vi "JKISM+ Worker Module.vi"(7 "Name":string="A") -> ()   [LabVIEW 2014]
uses:
  user.lib/_NEVSTOP/JKI State Machine ++/JKI-State-Machine-Plus.lvlib
panel:
  out "From Who":string
  out "Argument - State":string
  out "Arguments":string
  out "Current State":string
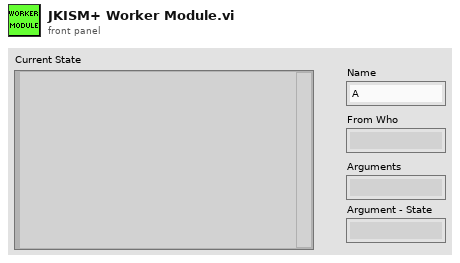
[diagram p1: front panel]
types:
  T1 = enum32{"Invalid", "Standard", "Closed", "Hidden", "Minimized", "Maximized"}
  T2 = enum32{"invalid app kind", "Development System", "Run Time System", "Student Edition", "Embedded LabVIEW", "Evaluation", "Custom"}
  T3 = cluster{"Core":cluster{"Current VI Reference":refnum<vi>, "Close Panel on Exit?":bool}, "Your Boolean data":bool, "Your string data":string}
  T4 = cluster{"Current VI Reference":refnum<vi>, "Close Panel on Exit?":bool}
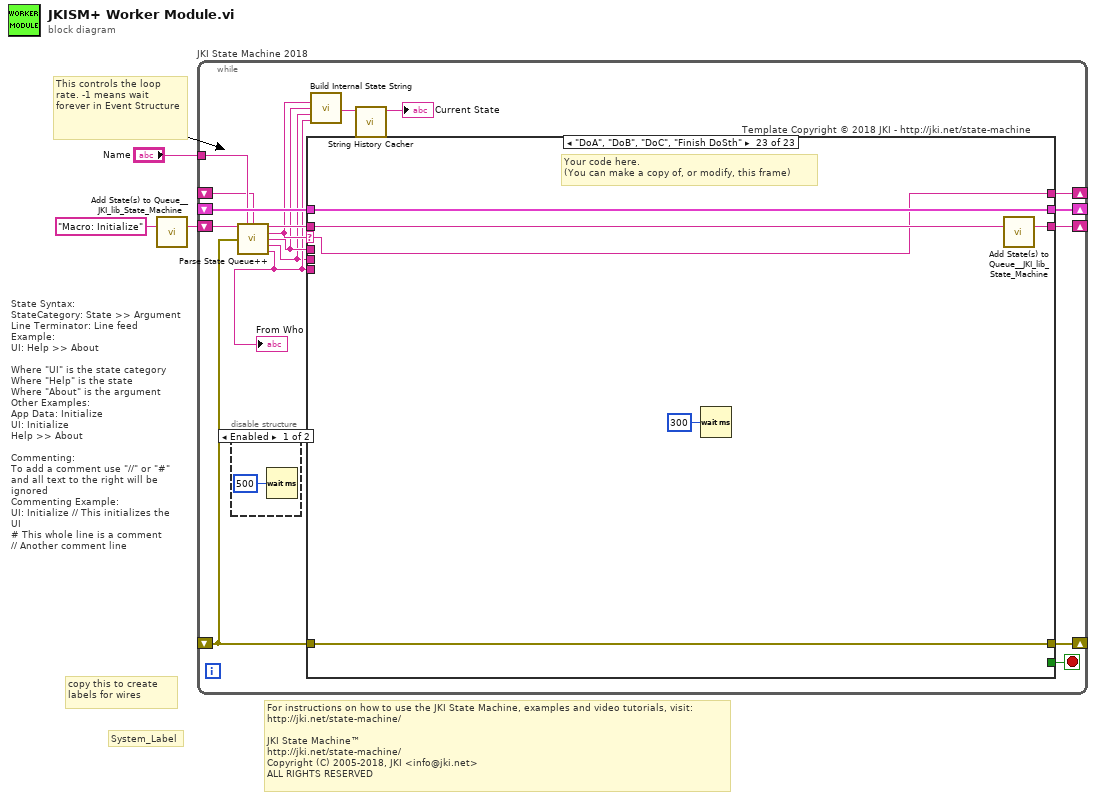
[diagram p0: block diagram]
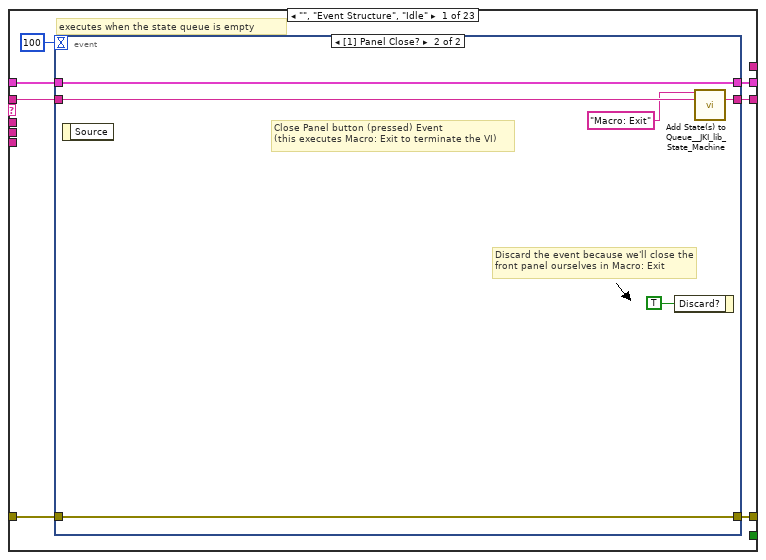
[diagram p3: hidden frame]
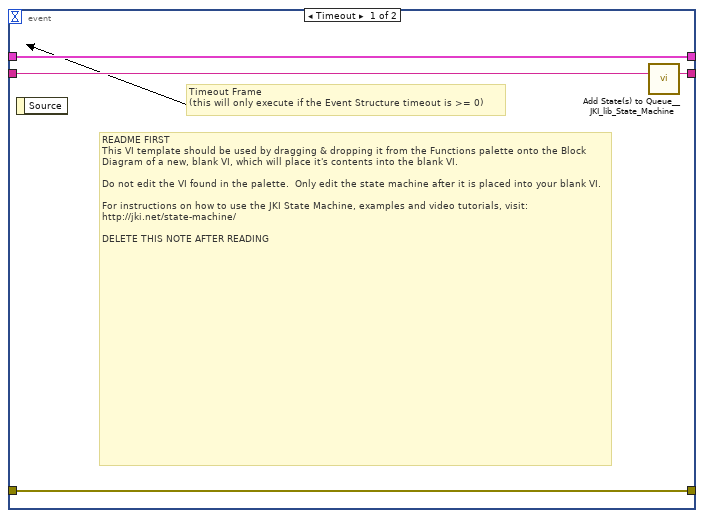
[diagram p4: hidden frame]
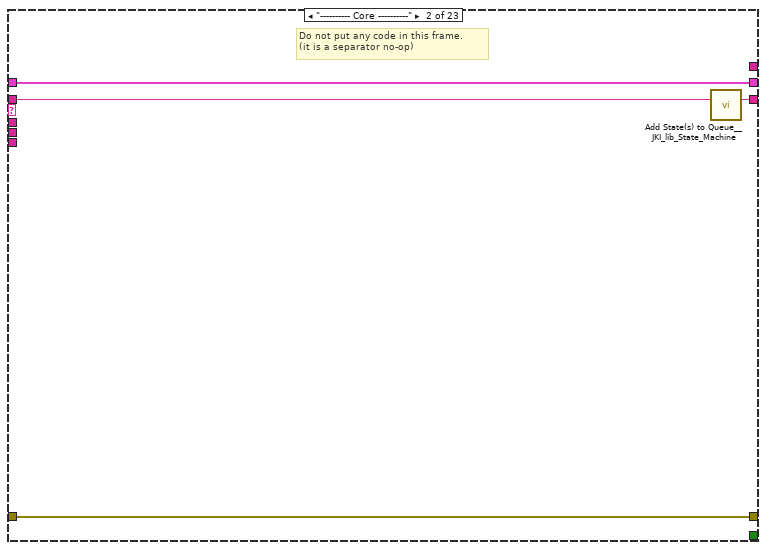
[diagram p5: hidden frame]
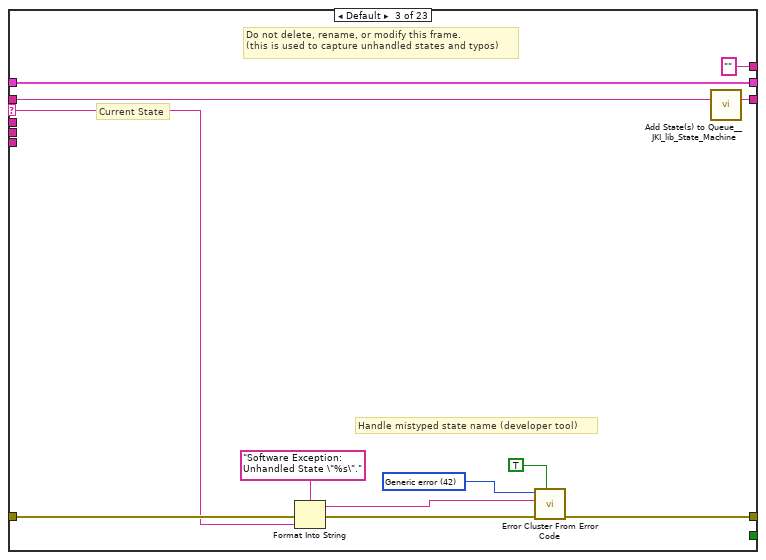
[diagram p6: hidden frame]
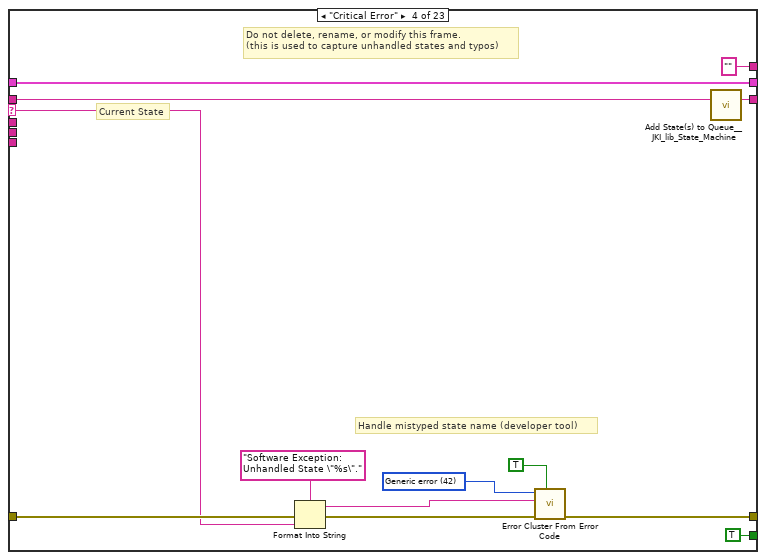
[diagram p7: hidden frame]
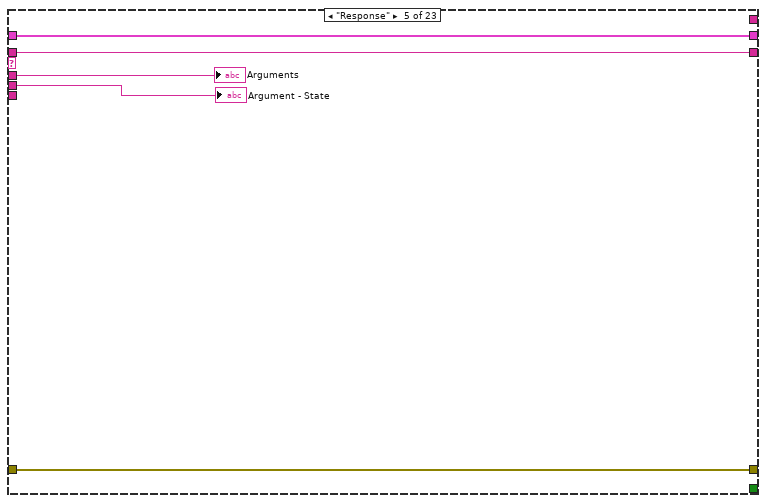
[diagram p8: hidden frame]
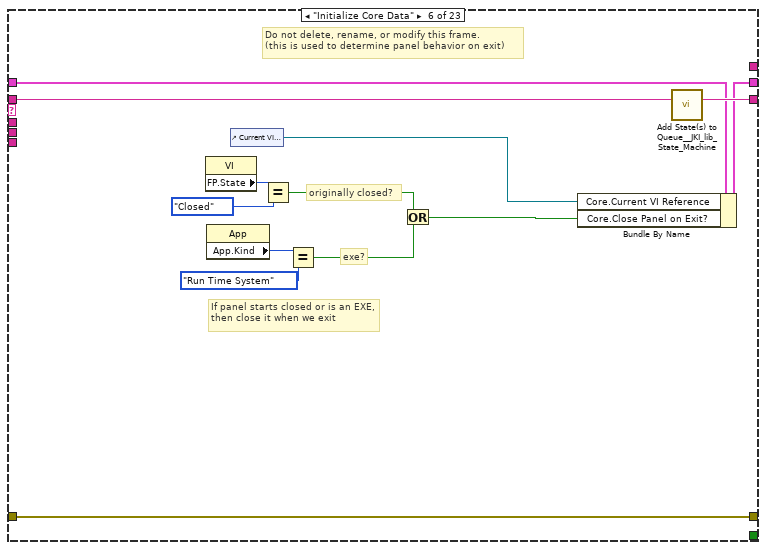
[diagram p9: hidden frame]
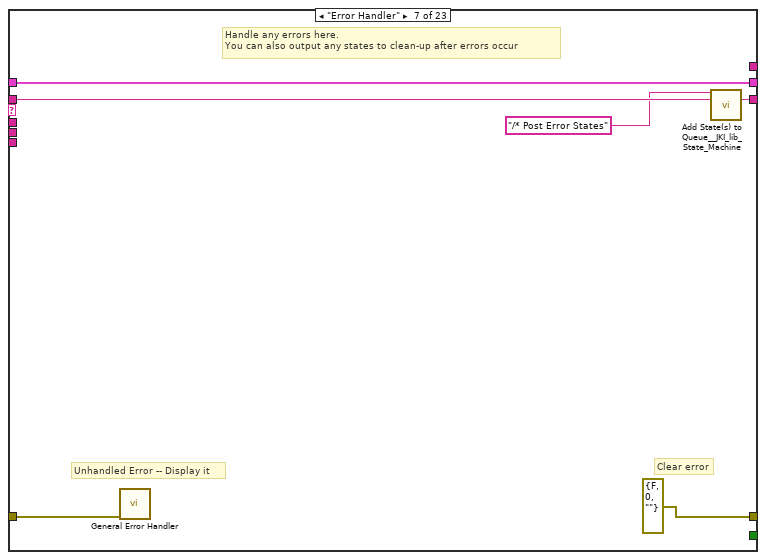
[diagram p10: hidden frame]
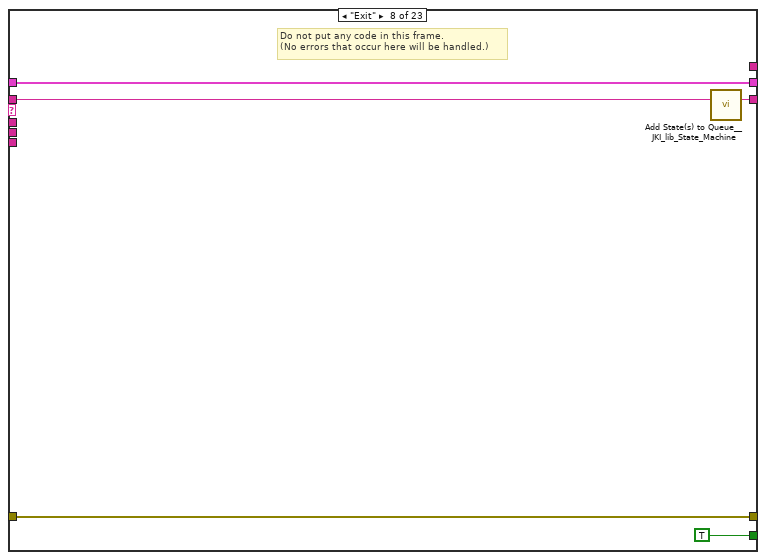
[diagram p11: hidden frame]
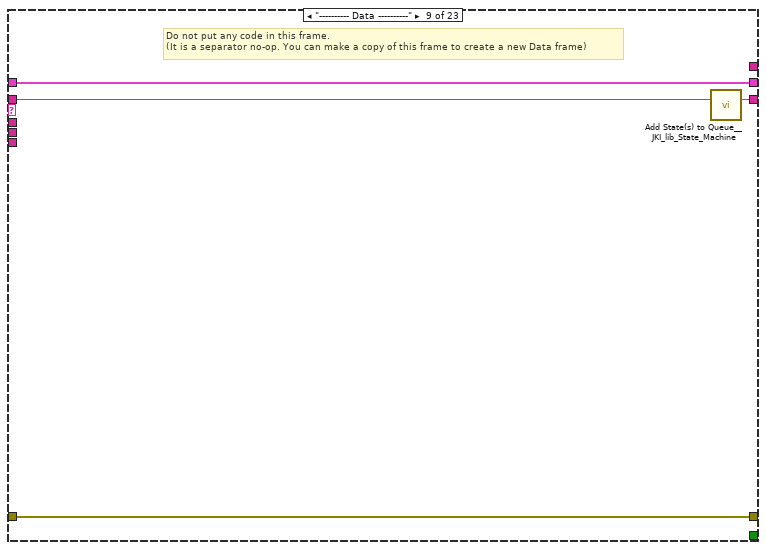
[diagram p12: hidden frame]
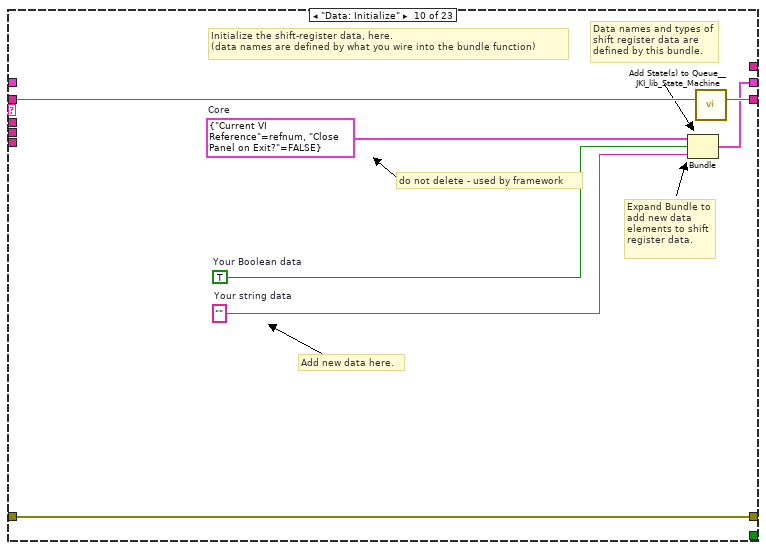
[diagram p13: hidden frame]
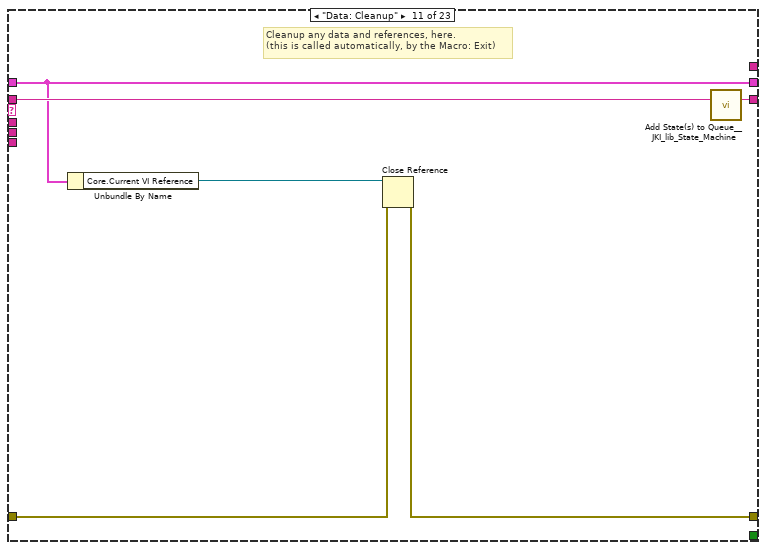
[diagram p14: hidden frame]
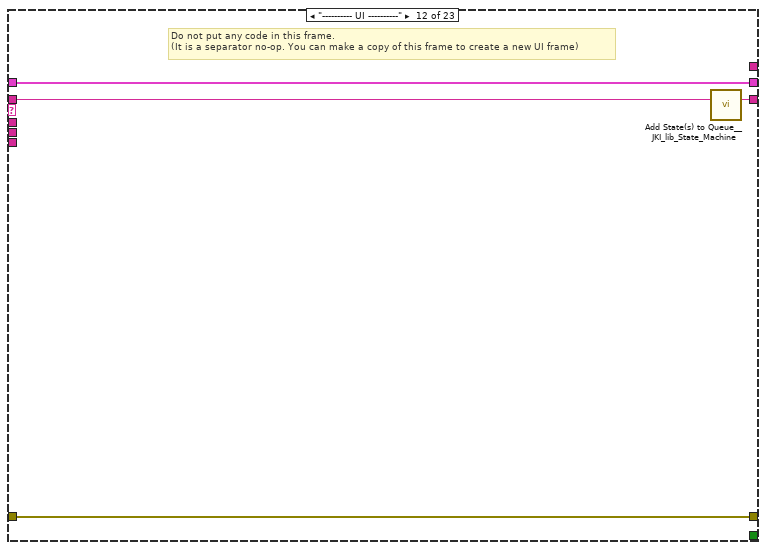
[diagram p15: hidden frame]
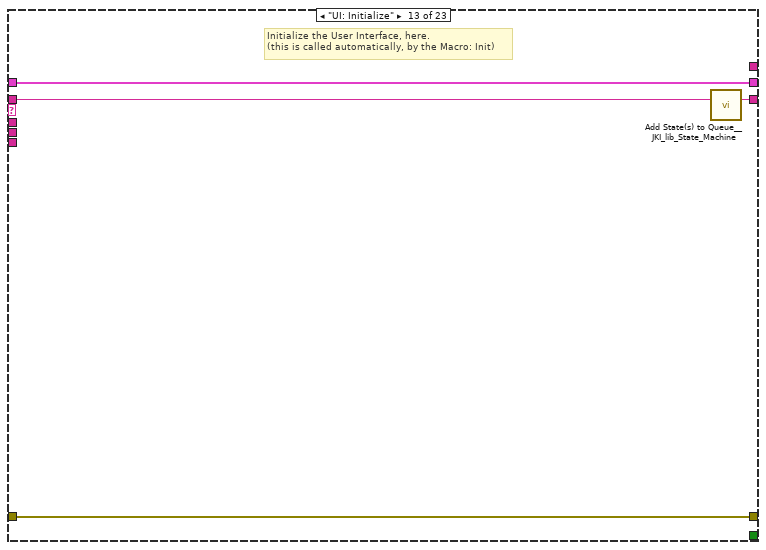
[diagram p16: hidden frame]
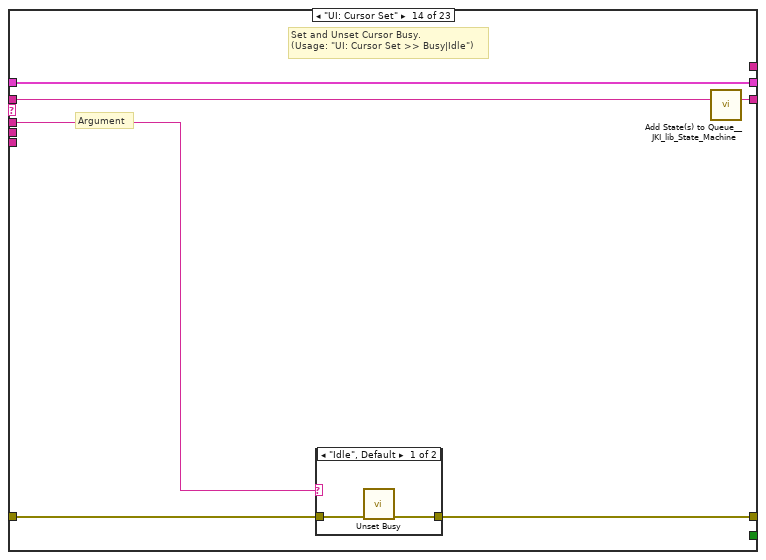
[diagram p17: hidden frame]
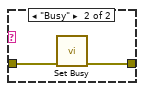
[diagram p18: hidden frame]
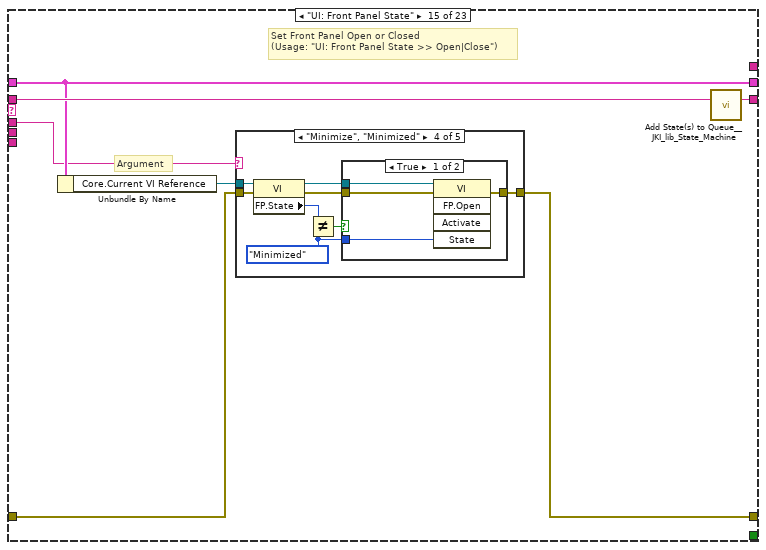
[diagram p19: hidden frame]
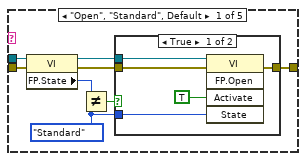
[diagram p20: hidden frame]
diagram:
  # "For instructions on how to use the JKI State Machine, examples and video tutorials, visit:\nhttp://jki.net/state-machine/\n\nJKI State Machine™\nhttp://jki.net/state-machine/\nCopyright (C) 2005-2018, JKI <info@jki.net>\nALL RIGHTS RESERVED"
  # "State Syntax:\nStateCategory: State >> Argument\nLine Terminator: Line feed\nExample:\nUI: Help >> About\n\nWhere \"UI\" is the state category\nWhere \"Help\" is the state\nWhere \"About\" is the argument\nOther Examples:\nApp Data: Initialize\nUI: Initialize\nHelp >> About\n\nCommenting:\nTo add a comment use \"//\" or \"#\" and all text to the right will be ignored\nCommenting Example:\nUI: Initialize // This initializes the UI\n# This whole line is a comment\n// Another comment line"
  # "copy this to create labels for wires"
  # "This controls the loop rate. -1 means wait forever in Event Structure"
  # "System_Label"
  n1 = call <vilib>:"Add State(s) to Queue__JKI_lib_State_Machine.vi"("State(s) in (\"\")"="Macro: Initialize") -> ("States Out"=w3:string)  [unwired: 14 in]
  n2 = while "JKI State Machine 2018" {
    shift-right: [w15] -> _
    shift-left: _ -> [w14]
    shift-right: [w18] -> _
    shift-left: _ -> [w13]
    shift-right: [w17] -> _
    shift-left: w3 -> [w19]
    tunnel: "Name" -> [w12]
    shift-right: [w5] -> _
    shift-left: _ -> [w4]
    stop <- w16 stop-if-true
    # "Template Copyright © 2018 JKI - http://jki.net/state-machine"
    n3 = disable-structure shown="Enabled" {
      frame Enabled {
        n4 = Wait (ms)(milliseconds to wait=u32 500) -> ()  [unwired: 1 out]
      }
      frame Disabled {
      }
    }
    n5 = call "Parse State Queue++.vi"("State Queue"=w19, "Name(\"\" to use uuid)"=w12, "Response Arguments"=w4, "Error In (no error)"=w13) -> ("Remaining States"=w20:string, "Current State"=w9:string, "Arguments"=w8:string, "Argument - State"=w6:string, "From Who"=w7:string)  [unwired: 7 in]
    "From Who" <- w7
    n6 = case shown="\"DoA\", \"DoB\", \"DoC\", \"Finish DoSth\"" w9 {
      selector: w9 -> [_ _ w44 w57 _ _ _ _ _ _ _ _ _ _ _ _ _ _ _ _ _ _ w240]
      tunnel: w20 -> [w28 w42 w48 w61 w72 w85 w91 w96 w100 w107 w113 w117 w121 w127 w138 w207 w212 w215 w227 w231 w235 w239 w245]
      tunnel: w8 -> [_ _ _ _ w69 _ _ _ _ _ _ _ _ w122 w132 _ _ _ _ _ _ _ _]
      tunnel: w14 -> [w26 w39 w46 w59 w71 w78 w88 w94 w97 _ w108 w114 w119 w125 w134 w204 w209 w217 w224 w228 w232 w236 w242]
      tunnel: [w25 w40 w50 w63 w70 w82 errorcluster {"status"=FALSE, "code"=0, "source"=""} ("error out") w93 w98 w104 w109 w115 w118 w123 w135 w205 w210 w213 w225 w229 w233 w237 w243] -> w18
      tunnel: w13 -> [w24 w40 w49 w62 w70 w82 w87 w93 w98 w104 w110 w115 w118 w124 w136 w205 w210 w213 w225 w229 w233 w237 w243]
      tunnel: [w27 w41 w47 w60 w72 w84 w90 w95 w99 w106 w112 w116 w120 w126 w137 w206 w211 w216 w226 w230 w234 w238 w244] -> w17
      tunnel: [_ _ _ TRUE _ _ _ TRUE _ _ _ _ _ _ _ _ _ _ _ _ _ _ _] -> w16
      tunnel: [w23 w39 w46 w59 w71 w83 w88 w94 w97 w105 w108 w114 w119 w125 w134 w204 w209 w217 w224 w228 w232 w236 w242] -> w15
      tunnel: w7 -> [_ _ _ _ _ _ _ _ _ _ _ _ _ _ _ _ _ _ _ _ _ _ _]
      tunnel: w6 -> [_ _ _ _ w68 _ _ _ _ _ _ _ _ _ _ _ _ _ _ _ _ _ _]
      tunnel: [_ _ "" ("Name") "" ("Name") _ _ _ _ _ _ _ _ _ _ _ _ _ _ _ _ _ _ w240] -> w5
      frame "", "Event Structure", "Idle" {
        # "executes when the state queue is empty"
        n7 = event shown="[1] Panel Close?" {
          selector: _ -> [_ _]
          dyn-events: _ -> [_ _]
          timeout: 100 ("Timeout") -> [_ _]
          tunnel: w28 -> [w32 w38]
          tunnel: [w31 w37] -> w27
          tunnel: w26 -> [w29 w35]
          tunnel: [w30 w36] -> w25
          tunnel: w24 -> [w30 w36]
          tunnel: [w29 w35] -> w23
          event Timeout {
            # "README FIRST\nThis VI template should be used by dragging & dropping it from the Functions palette onto the Block Diagram of a new, blank VI, which will place it's contents into the blank VI.\n\nDo not edit the VI found in the palette.  Only edit the state machine after it is placed into your blank VI.\n\nFor instructions on how to use the JKI State Machine, examples and video tutorials, visit:\nhttp://jki.net/state-machine/\n\nDELETE THIS NOTE AFTER READING"
            # "Timeout Frame\n(this will only execute if the Event Structure timeout is >= 0)"
            n8 = event-data() -> ()  [unwired: 1 in, 1 out]
            n9 = call <vilib>:"Add State(s) to Queue__JKI_lib_State_Machine.vi"("State(s) in (\"\")"=w32) -> ("States Out"=w31:string)  [unwired: 14 in]
          }
          event Panel Close? {
            # "Discard the event because we'll close the front panel ourselves in Macro: Exit"
            # "Close Panel button (pressed) Event\n(this executes Macro: Exit to terminate the VI)"
            n10 = event-data() -> ()  [unwired: 1 in, 1 out]
            n11 = event-data("Discard?"=TRUE) -> ()  [unwired: 1 in, 1 out]
            n12 = call <vilib>:"Add State(s) to Queue__JKI_lib_State_Machine.vi"("State(s) in Front (\"\")"="Macro: Exit", "State(s) in (\"\")"=w38) -> ("States Out"=w37:string)  [unwired: 13 in]
          }
        }
      }
      frame "---------- Core ----------" {
        # "Do not put any code in this frame.\n(it is a separator no-op)"
        n13 = call <vilib>:"Add State(s) to Queue__JKI_lib_State_Machine.vi"("State(s) in (\"\")"=w42) -> ("States Out"=w41:string)  [unwired: 14 in]
      }
      frame Default {
        w53 = 42 items=["No error", "Argument error", "Memory is full", "Out of zone", "End of file", "File already open", "Generic file I/O error", "File not found", "File permission error", "Disk is full", "Duplicate path", "Too many files open", "System feature not enabled", "Resource file not found", "Cannot add resource", "Resource not found", "Image not found", "Image memory error", "Pen does not exist", "Config type invalid", "Config token not found", "Config parse error", "Config memory error", "Bad external code format", "Bad external code offset", "External code not present", "Null window", "Destroy window error", "Null menu", "Print aborted", "Bad print record", "Print driver error", "Windows error during printing", "Memory error during printing", "Print dialog error", "Generic print error", "Invalid device refnum", "Device not found", "Device parameter error", "Device unit error", "Cannot open device", "Device call aborted", "Generic error", "Cancelled by user", "Object ID too low", "Object ID too high", "Object not in heap", "Unknown heap", "Unknown object (invalid DefProc)", "Unknown object (DefProc not in table)", "Message out of range", "Invalid (null) method", "Unknown message", "Manager call not supported", "Bad address", "Network operation in progress", "Network operation timed out", "Connection is busy", "Network attribute not supported", "Network error", "Address in use", "System out of memory", "Connection aborted", "Connection refused", "Not connected", "Already connected", "Connection closed", "Initialization error (interapplication manager)", "Bad occurrence", "Wait on unbound occurrence handler", "Occurrence queue overflow", "Datalog type conflict", "Unused", "Unrecognized type (interapplication manager)", "Memory corrupt", "Failed to make temporary DLL", "Old CIN version", "Drag socket not found", "Failed to load drop-object", "Failed to register OLE object", "Failed to release OLE object", "Format specifier type mismatch", "Unknown format specifier", "Too few format specifiers", "Too many format specifiers", "Scan failed", "Newer CIN version", "Error converting to variant", "Runtime menu error", "Password tampered", "Variant attribute not found", "Incompatible variant data type", "Event data is not available", "Event Store is not present", "Occurrence is not found", "Event Queue is not created", "Event info is not available", "Refnum passed is NULL", "Error retrieving Class GUID", "Error retrieving CoClass GUID", "Error retrieving TypeLib GUID.", "Bad built application magic bytes.", "Specific driver is different from the specific driver associated with the Logical Name.", "There is no session opened to the class driver.", "Max Error", "MAX - Error with config objects", "MAX - Error loading configuration", "MAX - Group not supported"]
        # "Current State"
        # "Do not delete, rename, or modify this frame.\n(this is used to capture unhandled states and typos)"
        # "Handle mistyped state name (developer tool)"
        n14 = Format Into String(format string="Software Exception: Unhandled State \"%s\"." ("message"), error in=w49, w44) -> (resulting string=w52:string, error out=w51:errorcluster)  [unwired: 1 in]
        n15 = call <vilib>:"Error Cluster From Error Code.vi"("show call chain? (False)"=TRUE, "error in (no error)"=w51, "error message (\"\")"=w52, "error code (0)"=w53) -> ("error out"=w50:errorcluster)  [unwired: 5 in]
        n16 = call <vilib>:"Add State(s) to Queue__JKI_lib_State_Machine.vi"("State(s) in (\"\")"=w48) -> ("States Out"=w47:string)  [unwired: 14 in]
      }
      frame "Critical Error" {
        w66 = 42 items=["No error", "Argument error", "Memory is full", "Out of zone", "End of file", "File already open", "Generic file I/O error", "File not found", "File permission error", "Disk is full", "Duplicate path", "Too many files open", "System feature not enabled", "Resource file not found", "Cannot add resource", "Resource not found", "Image not found", "Image memory error", "Pen does not exist", "Config type invalid", "Config token not found", "Config parse error", "Config memory error", "Bad external code format", "Bad external code offset", "External code not present", "Null window", "Destroy window error", "Null menu", "Print aborted", "Bad print record", "Print driver error", "Windows error during printing", "Memory error during printing", "Print dialog error", "Generic print error", "Invalid device refnum", "Device not found", "Device parameter error", "Device unit error", "Cannot open device", "Device call aborted", "Generic error", "Cancelled by user", "Object ID too low", "Object ID too high", "Object not in heap", "Unknown heap", "Unknown object (invalid DefProc)", "Unknown object (DefProc not in table)", "Message out of range", "Invalid (null) method", "Unknown message", "Manager call not supported", "Bad address", "Network operation in progress", "Network operation timed out", "Connection is busy", "Network attribute not supported", "Network error", "Address in use", "System out of memory", "Connection aborted", "Connection refused", "Not connected", "Already connected", "Connection closed", "Initialization error (interapplication manager)", "Bad occurrence", "Wait on unbound occurrence handler", "Occurrence queue overflow", "Datalog type conflict", "Unused", "Unrecognized type (interapplication manager)", "Memory corrupt", "Failed to make temporary DLL", "Old CIN version", "Drag socket not found", "Failed to load drop-object", "Failed to register OLE object", "Failed to release OLE object", "Format specifier type mismatch", "Unknown format specifier", "Too few format specifiers", "Too many format specifiers", "Scan failed", "Newer CIN version", "Error converting to variant", "Runtime menu error", "Password tampered", "Variant attribute not found", "Incompatible variant data type", "Event data is not available", "Event Store is not present", "Occurrence is not found", "Event Queue is not created", "Event info is not available", "Refnum passed is NULL", "Error retrieving Class GUID", "Error retrieving CoClass GUID", "Error retrieving TypeLib GUID.", "Bad built application magic bytes.", "Specific driver is different from the specific driver associated with the Logical Name.", "There is no session opened to the class driver.", "Max Error", "MAX - Error with config objects", "MAX - Error loading configuration", "MAX - Group not supported"]
        # "Current State"
        # "Do not delete, rename, or modify this frame.\n(this is used to capture unhandled states and typos)"
        # "Handle mistyped state name (developer tool)"
        n17 = Format Into String(format string="Software Exception: Unhandled State \"%s\"." ("message"), error in=w62, w57) -> (resulting string=w65:string, error out=w64:errorcluster)  [unwired: 1 in]
        n18 = call <vilib>:"Error Cluster From Error Code.vi"("show call chain? (False)"=TRUE, "error in (no error)"=w64, "error message (\"\")"=w65, "error code (0)"=w66) -> ("error out"=w63:errorcluster)  [unwired: 5 in]
        n19 = call <vilib>:"Add State(s) to Queue__JKI_lib_State_Machine.vi"("State(s) in (\"\")"=w61) -> ("States Out"=w60:string)  [unwired: 14 in]
      }
      frame "Response" {
        "Arguments" <- w69
        "Argument - State" <- w68
      }
      frame "Initialize Core Data" {
        # "Do not delete, rename, or modify this frame.\n(this is used to determine panel behavior on exit)"
        # "originally closed?"
        # "exe?"
        # "If panel starts closed or is an EXE, then close it when we exit"
        n20 = property class="VI"() -> ("FP.State"=w75:T1)  [unwired: 2 in, 2 out]
        n21 = property class="App"() -> ("App.Kind"=w81:T2)  [unwired: 2 in, 2 out]
        n22 = control-ref of="Current VI Reference"() -> (w76:refnum<vi>)
        n23 = Equal?(x=w75, y=T1."Closed" ("Front Panel Window:State")) -> (x = y?=w73:bool)
        n24 = Equal?(x=w81, y=T2."Run Time System" ("Application:Kind")) -> (x = y?=w79:bool)
        n25 = Or(x=w73, y=w79) -> (x .or. y?=w77:bool)
        n26 = Bundle By Name(cluster=w78, "Core.Current VI Reference"=w76, "Core.Close Panel on Exit?"=w77) -> (w83:T3)
        n27 = call <vilib>:"Add State(s) to Queue__JKI_lib_State_Machine.vi"("State(s) in (\"\")"=w85) -> ("States Out"=w84:string)  [unwired: 14 in]
      }
      frame "Error Handler" {
        # "Unhandled Error -- Display it"
        # "Handle any errors here.\nYou can also output any states to clean-up after errors occur"
        # "Clear error"
        n28 = call <vilib>:"General Error Handler.vi"("error in (no error)"=w87) -> ()  [unwired: 10 in, 5 out]
        n29 = call <vilib>:"Add State(s) to Queue__JKI_lib_State_Machine.vi"("State(s) in Front (\"\")"="/* Post Error States", "State(s) in (\"\")"=w91) -> ("States Out"=w90:string)  [unwired: 13 in]
      }
      frame "Exit" {
        # "Do not put any code in this frame.\n(No errors that occur here will be handled.)"
        n30 = call <vilib>:"Add State(s) to Queue__JKI_lib_State_Machine.vi"("State(s) in (\"\")"=w96) -> ("States Out"=w95:string)  [unwired: 14 in]
      }
      frame "---------- Data ----------" {
        # "Do not put any code in this frame.\n(It is a separator no-op. You can make a copy of this frame to create a new Data frame)"
        n31 = call <vilib>:"Add State(s) to Queue__JKI_lib_State_Machine.vi"("State(s) in (\"\")"=w100) -> ("States Out"=w99:string)  [unwired: 14 in]
      }
      frame "Data: Initialize" {
        w101 = T4 {"Current VI Reference"=refnum, "Close Panel on Exit?"=FALSE}  # Core
        w103 = TRUE  # Your Boolean data
        w102 = ""  # Your string data
        # "do not delete - used by framework"
        # "Expand Bundle to add new data elements to shift register data."
        # "Add new data here."
        # "Data names and types of shift register data are defined by this bundle."
        # "Initialize the shift-register data, here.\n(data names are defined by what you wire into the bundle function)"
        n32 = Bundle("Core"=w101, "Your Boolean data"=w103, "Your string data"=w102) -> (w105:T3)  [unwired: 1 in]
        n33 = call <vilib>:"Add State(s) to Queue__JKI_lib_State_Machine.vi"("State(s) in (\"\")"=w107) -> ("States Out"=w106:string)  [unwired: 14 in]
      }
      frame "Data: Cleanup" {
        # "Cleanup any data and references, here.\n(this is called automatically, by the Macro: Exit)"
        n34 = Unbundle By Name(w108) -> ("Core.Current VI Reference"=w111:refnum<vi>)
        n35 = Close Reference(reference=w111, error in (no error)=w110) -> (error out=w109:errorcluster)
        n36 = call <vilib>:"Add State(s) to Queue__JKI_lib_State_Machine.vi"("State(s) in (\"\")"=w113) -> ("States Out"=w112:string)  [unwired: 14 in]
      }
      frame "---------- UI ----------" {
        # "Do not put any code in this frame.\n(It is a separator no-op. You can make a copy of this frame to create a new UI frame)"
        n37 = call <vilib>:"Add State(s) to Queue__JKI_lib_State_Machine.vi"("State(s) in (\"\")"=w117) -> ("States Out"=w116:string)  [unwired: 14 in]
      }
      frame "UI: Initialize" {
        # "Initialize the User Interface, here.\n(this is called automatically, by the Macro: Init)"
        n38 = call <vilib>:"Add State(s) to Queue__JKI_lib_State_Machine.vi"("State(s) in (\"\")"=w121) -> ("States Out"=w120:string)  [unwired: 14 in]
      }
      frame "UI: Cursor Set" {
        # "Argument"
        # "Set and Unset Cursor Busy.\n(Usage: \"UI: Cursor Set >> Busy|Idle\")"
        n39 = case shown="\"Idle\", Default" w122 {
          tunnel: w124 -> [w129 w131]
          tunnel: [w128 w130] -> w123
          frame "Idle", Default {
            n40 = call <vilib>:"Unset Busy.vi"("error in (no error)"=w129) -> ("error out"=w128:errorcluster)  [unwired: 10 in]
          }
          frame "Busy" {
            n41 = call <vilib>:"Set Busy.vi"("error in (no error)"=w131) -> ("error out"=w130:errorcluster)  [unwired: 9 in, 1 out]
          }
        }
        n42 = call <vilib>:"Add State(s) to Queue__JKI_lib_State_Machine.vi"("State(s) in (\"\")"=w127) -> ("States Out"=w126:string)  [unwired: 14 in]
      }
      frame "UI: Front Panel State" {
        # "Argument"
        # "Set Front Panel Open or Closed\n(Usage: \"UI: Front Panel State >> Open|Close\")"
        n43 = Unbundle By Name(w134) -> ("Core.Current VI Reference"=w133:refnum<vi>)
        n44 = case shown="\"Minimize\", \"Minimized\"" w132 {
          tunnel: w136 -> [w144 w159 w170 w183 w196]
          tunnel: [w146 w160 w172 w185 w198] -> w135
          tunnel: w133 -> [w145 w157 w171 w184 w197]
          frame "Open", "Standard", Default {
            w139 = T1."Standard" ("State")
            n45 = property class="VI"(reference=w145, error in=w144) -> (reference out=w142:refnum<vi>, error out=w143:errorcluster, "FP.State"=w141:T1)
            n46 = Not Equal?(x=w141, y=w139) -> (x != y?=w140:bool)
            n47 = case shown="True" w140 {
              tunnel: [w150 w152] -> w146
              tunnel: w143 -> [w149 w152]
              tunnel: w142 -> [w148 _]
              tunnel: w139 -> [w147 _]
              frame True {
                n48 = invoke class="VI" method="FP.Open"(reference=w148, error in=w149, "Activate"=TRUE, "State"=w147) -> (error out=w150:errorcluster)  [unwired: 1 in, 4 out]
              }
              frame False {
              }
            }
          }
          frame "Close", "Closed" {
            n49 = property class="VI"(reference=w157, error in=w159) -> (reference out=w156:refnum<vi>, error out=w158:errorcluster, "FP.State"=w154:T1)
            n50 = Not Equal?(x=w154, y=T1."Closed" ("Front Panel Window:State")) -> (x != y?=w153:bool)
            n51 = case shown="True" w153 {
              tunnel: [w161 w164] -> w160
              tunnel: w158 -> [w161 w163]
              tunnel: w156 -> [_ w162]
              frame False {
              }
              frame True {
                n52 = invoke class="VI" method="FP.Close"(reference=w162, error in=w163) -> (error out=w164:errorcluster)  [unwired: 1 in, 2 out]
              }
            }
          }
          frame "Hidden", "Hide" {
            w165 = T1."Hidden" ("State")
            n53 = property class="VI"(reference=w171, error in=w170) -> (reference out=w168:refnum<vi>, error out=w169:errorcluster, "FP.State"=w167:T1)
            n54 = Not Equal?(x=w167, y=w165) -> (x != y?=w166:bool)
            n55 = case shown="True" w166 {
              tunnel: [w176 w177] -> w172
              tunnel: w169 -> [w175 w177]
              tunnel: w168 -> [w174 _]
              tunnel: w165 -> [w173 _]
              frame True {
                n56 = invoke class="VI" method="FP.Open"(reference=w174, error in=w175, "State"=w173) -> (error out=w176:errorcluster)  [unwired: 2 in, 4 out]
              }
              frame False {
              }
            }
          }
          frame "Minimize", "Minimized" {
            w178 = T1."Minimized" ("State")
            n57 = property class="VI"(reference=w184, error in=w183) -> (reference out=w181:refnum<vi>, error out=w182:errorcluster, "FP.State"=w180:T1)
            n58 = Not Equal?(x=w180, y=w178) -> (x != y?=w179:bool)
            n59 = case shown="True" w179 {
              tunnel: [w189 w190] -> w185
              tunnel: w182 -> [w188 w190]
              tunnel: w181 -> [w187 _]
              tunnel: w178 -> [w186 _]
              frame True {
                n60 = invoke class="VI" method="FP.Open"(reference=w187, error in=w188, "State"=w186) -> (error out=w189:errorcluster)  [unwired: 2 in, 4 out]
              }
              frame False {
              }
            }
          }
          frame "Maximize", "Maximized" {
            w191 = T1."Maximized" ("State")
            n61 = property class="VI"(reference=w197, error in=w196) -> (reference out=w194:refnum<vi>, error out=w195:errorcluster, "FP.State"=w193:T1)
            n62 = Not Equal?(x=w193, y=w191) -> (x != y?=w192:bool)
            n63 = case shown="True" w192 {
              tunnel: [w202 w203] -> w198
              tunnel: w195 -> [w201 w203]
              tunnel: w194 -> [w200 _]
              tunnel: w191 -> [w199 _]
              frame True {
                n64 = invoke class="VI" method="FP.Open"(reference=w200, error in=w201, "State"=w199) -> (error out=w202:errorcluster)  [unwired: 2 in, 4 out]
              }
              frame False {
              }
            }
          }
        }
        n65 = call <vilib>:"Add State(s) to Queue__JKI_lib_State_Machine.vi"("State(s) in (\"\")"=w138) -> ("States Out"=w137:string)  [unwired: 14 in]
      }
      frame "---------- Macro ----------" {
        # "Do not put any code in this frame.\n(It is a separator no-op. You can make a copy of this frame to create a new Macro frame)"
        n66 = call <vilib>:"Add State(s) to Queue__JKI_lib_State_Machine.vi"("State(s) in (\"\")"=w207) -> ("States Out"=w206:string)  [unwired: 14 in]
      }
      frame "Macro: Initialize" {
        w208 = "Data: Initialize\nInitialize Core Data\nUI: Initialize\nUI: Front Panel State >> Open"  # Data: Initialize Initialize Core Data UI: Initialize UI: Front Panel State >> Open
        # "Initialization Macro\n(This is called once, when the VI starts)"
        n67 = call <vilib>:"Add State(s) to Queue__JKI_lib_State_Machine.vi"("State(s) in Front (\"\")"=w208, "State(s) in (\"\")"=w212) -> ("States Out"=w211:string)  [unwired: 13 in]
      }
      frame "Macro: DoSth" {
        n68 = call <vilib>:"Add State(s) to Queue__JKI_lib_State_Machine.vi"("State(s) in Front (\"\")"="DoA\nDoB\nDoC\nFinish DoSth" ("State(s) in Front (\"\")"), "State(s) in (\"\")"=w215) -> ("States Out"=w216:string)  [unwired: 13 in]
      }
      frame "Macro: Exit" {
        # "Exit Macro\n(This is called once, when the VI exits)"
        n69 = Unbundle By Name(w224) -> ("Core.Close Panel on Exit?"=w223:bool)
        n70 = Select(t="UI: Front Panel State >> Close", s=w223, f="") -> (s? t:f=w220:string)
        n71 = call <vilib>:"Add State(s) to Queue__JKI_lib_State_Machine.vi"("State(s) in (\"\")"=w220, "State(s) at Back (\"\")"="Data: Cleanup\nExit") -> ("States Out"=w218:string)  [unwired: 13 in]
        n72 = call <vilib>:"Add State(s) to Queue__JKI_lib_State_Machine.vi"("State(s) in Front (\"\")"=w218, "State(s) in (\"\")"=w227) -> ("States Out"=w226:string)  [unwired: 13 in]
      }
      frame "---------- New Category ----------" {
        # "Template Separator\n(You can make a copy of, or modify, this frame)"
        n73 = call <vilib>:"Add State(s) to Queue__JKI_lib_State_Machine.vi"("State(s) in (\"\")"=w231) -> ("States Out"=w230:string)  [unwired: 14 in]
      }
      frame "New Category: 1" {
        # "Your code here.\n(You can make a copy of, or modify, this frame)"
        n74 = call <vilib>:"Add State(s) to Queue__JKI_lib_State_Machine.vi"("State(s) in (\"\")"=w235) -> ("States Out"=w234:string)  [unwired: 14 in]
      }
      frame "New Category: 2" {
        # "Your code here.\n(You can make a copy of, or modify, this frame)"
        n75 = call <vilib>:"Add State(s) to Queue__JKI_lib_State_Machine.vi"("State(s) in (\"\")"=w239) -> ("States Out"=w238:string)  [unwired: 14 in]
      }
      frame "DoA", "DoB", "DoC", "Finish DoSth" {
        # "Your code here.\n(You can make a copy of, or modify, this frame)"
        n76 = Wait (ms)(milliseconds to wait=u32 300) -> ()  [unwired: 1 out]
        n77 = call <vilib>:"Add State(s) to Queue__JKI_lib_State_Machine.vi"("State(s) in (\"\")"=w245) -> ("States Out"=w244:string)  [unwired: 14 in]
      }
    }
    n78 = call "Build Internal State String.vi"("State"=w9, "Arguments (\"\")"=w8, "Arg-State (\"\")"=w6, "Source (\"\")"=w7) -> ("State with Arguments"=w10:string)  [unwired: 11 in]
    n79 = call "String History Cacher.vi"("String"=w10) -> ("String Cache"=→"Current State":string)  [unwired: 10 in]
  }
